vi "Synchronize Scroll.vi"(8 "error in (no error)":errorcluster, 9 "Direction":T1, 10 "Other 2D Array":refnum<class "2DArrayManager.lvclass">, 11 "2DArrayManager in":refnum<class "2DArrayManager.lvclass">) -> (0 "error out":errorcluster, 3 "2DArrayManager out":refnum<class "2DArrayManager.lvclass">)   [LabVIEW 2020, in "OOPanel.lvlib" / "2DArrayManager.lvclass"]
uses:
  2DArrayManager.lvclass
  Direction.ctl
  OOPanel.lvlib
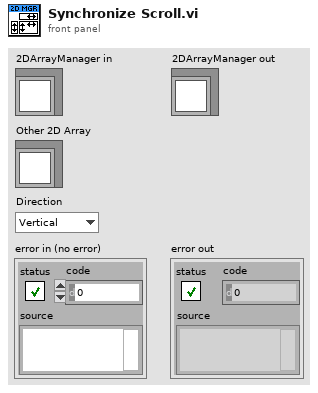
[diagram p1: front panel]
types:
  T1 = typedef "OOPanel.lvlib/Direction.ctl" = enum16{"Vertical", "Horizontal", "Both"}
  T2 = typedef "OOPanel.lvlib/2DArrayManager.lvclass/State.ctl" = cluster{"Scroll":T3, "Scroll Max":T3, "Top-Left Index":T4, "H Scroll Sync":refnum<user-event>, "V Scroll Sync":refnum<user-event>, "Sync":bool, "H Scroll Vis":bool, "V Scroll Vis":bool, "Blank Pool":refnum<queue>}
  T3 = typedef "OOPanel.lvlib/2D Position.ctl" = cluster{"H":i32, "V":i32}
  T4 = typedef "OOPanel.lvlib/2D Index.ctl" = cluster{"Row":i32, "Col":i32}
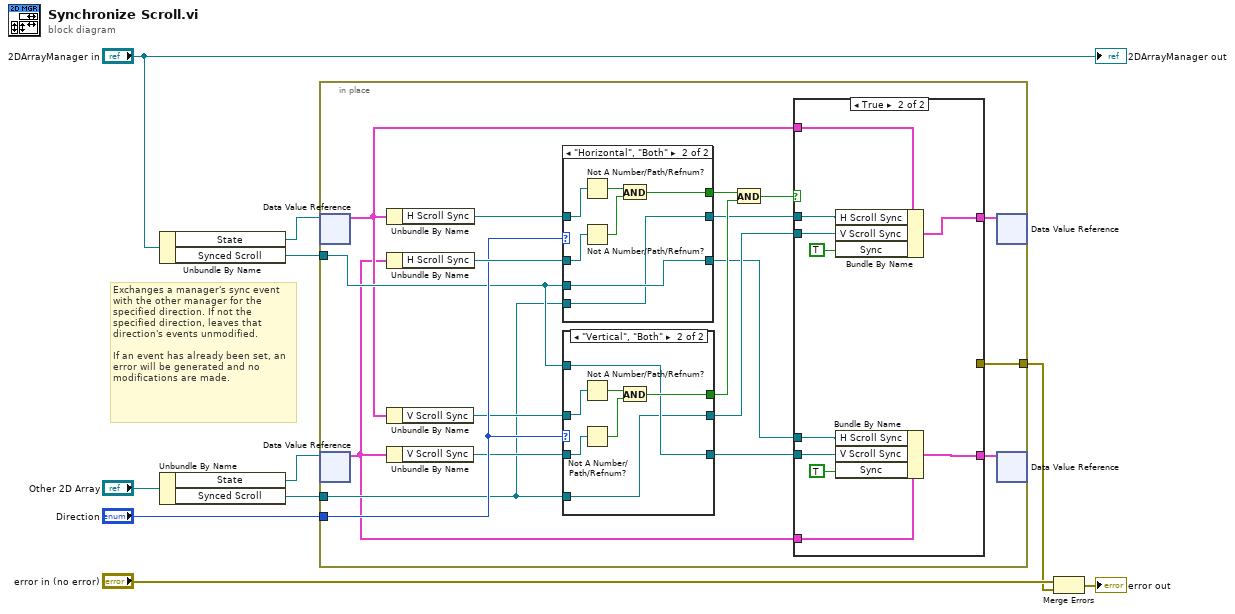
[diagram p0: block diagram]
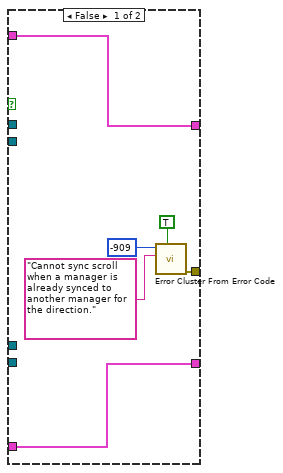
[diagram p2: hidden frame]
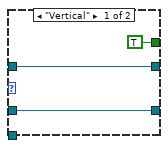
[diagram p3: hidden frame]
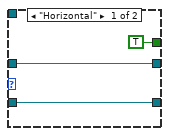
[diagram p4: hidden frame]
diagram:
  # "Exchanges a manager's sync event with the other manager for the specified direction. If not the specified direction, leaves that direction's events unmodified.\n\nIf an event has already been set, an error will be generated and no modifications are made."
  n1 = Unbundle By Name("2DArrayManager in") -> ("State"=w6:refnum<data-value>, "Synced Scroll"=w5:refnum<user-event>)
  n2 = Unbundle By Name("Other 2D Array") -> ("State"=w7:refnum<data-value>, "Synced Scroll"=w4:refnum<user-event>)
  n3 = in-place {
    in-place-border: w5 -> [w24]
    in-place-border: w4 -> [w21]
    in-place-border: "Direction" -> [w27]
    in-place-border: [w11] -> w1
    n4 = in-place-dvr #1(w6) -> (w20:T2)  [unwired: 1 out]
    n5 = in-place-dvr #2(w7) -> (w15:T2)  [unwired: 1 out]
    n6 = Unbundle By Name(w20) -> ("H Scroll Sync"=w28:refnum<user-event>)
    n7 = Unbundle By Name(w15) -> ("H Scroll Sync"=w29:refnum<user-event>)
    n8 = Unbundle By Name(w20) -> ("V Scroll Sync"=w26:refnum<user-event>)
    n9 = Unbundle By Name(w15) -> ("V Scroll Sync"=w25:refnum<user-event>)
    n10 = case shown="\"Horizontal\", \"Both\"" w27 {
      tunnel: w29 -> [w47 w54]
      tunnel: w28 -> [w48 w55]
      tunnel: [w48 w49] -> w19
      tunnel: [w47 w50] -> w16
      tunnel: w24 -> [_ w50]
      tunnel: [TRUE w51] -> w23
      tunnel: w21 -> [_ w49]
      frame "Vertical" {
      }
      frame "Horizontal", "Both" {
        n11 = Not A Number/Path/Refnum?(number/path/refnum=w55) -> (NaN/Path/Refnum?=w53:bool)
        n12 = Not A Number/Path/Refnum?(number/path/refnum=w54) -> (NaN/Path/Refnum?=w52:bool)
        n13 = And(x=w53, y=w52) -> (x .and. y?=w51:bool)
      }
    }
    n14 = case shown="\"Vertical\", \"Both\"" w27 {
      tunnel: w26 -> [w57 w65]
      tunnel: [w58 w60] -> w17
      tunnel: w25 -> [w58 w64]
      tunnel: [w57 w59] -> w18
      tunnel: w21 -> [_ w59]
      tunnel: w24 -> [_ w60]
      tunnel: [TRUE w61] -> w22
      frame "Horizontal" {
      }
      frame "Vertical", "Both" {
        n15 = Not A Number/Path/Refnum?(number/path/refnum=w65) -> (NaN/Path/Refnum?=w63:bool)
        n16 = Not A Number/Path/Refnum?(number/path/refnum=w64) -> (NaN/Path/Refnum?=w62:bool)
        n17 = And(x=w63, y=w62) -> (x .and. y?=w61:bool)
      }
    }
    n18 = And(x=w23, y=w22) -> (x .and. y?=w12:bool)
    n19 = case shown="True" w12 {
      tunnel: w20 -> [w34 w45]
      tunnel: w19 -> [_ w44]
      tunnel: w18 -> [_ w43]
      tunnel: w17 -> [_ w42]
      tunnel: w16 -> [_ w41]
      tunnel: w15 -> [w35 w40]
      tunnel: [w35 w39] -> w14
      tunnel: [w34 w38] -> w13
      tunnel: [w30 _] -> w11
      frame False {
        n20 = call <vilib>:"Error Cluster From Error Code.vi"("show call chain? (False)"=TRUE, "error message (\"\")"="Cannot sync scroll when a manager is already synced to another manager for the direction." ("error message (\"\")"), "error code (0)"=-909) -> ("error out"=w30:errorcluster)  [unwired: 6 in]
      }
      frame True {
        n21 = Bundle By Name(cluster=w45, "H Scroll Sync"=w44, "V Scroll Sync"=w43, "Sync"=TRUE) -> (w38:T2)
        n22 = Bundle By Name(cluster=w40, "H Scroll Sync"=w41, "V Scroll Sync"=w42, "Sync"=TRUE) -> (w39:T2)
      }
    }
    n23 = in-place-dvr #1(w13) -> ()  [unwired: 2 out]
    n24 = in-place-dvr #2(w14) -> ()  [unwired: 2 out]
  }
  n25 = Merge Errors("error in (no error)", w1) -> (→"error out":errorcluster)
  "2DArrayManager out" <- "2DArrayManager in"
